vi "ex_GetPacketData.vi"(0 "file refs":T1={"file ref"=refnum, "file size (bytes:0)"=0, "read pointer (bytes:0)"=0, "chunk size (bytes:65000)"=65000}, 1 "channel info in":T3[](array[typedef]) {"Delta X" format="%.2p"; "X0" format="%<%X\n%x>T"; "Timestamp" format="%<%X\n%x>T"}, 2 "first call?":bool=TRUE, 5 "current chunk":string, 7 "delimiter":string="\t", 9 "file_params":T2={"include col headings?"=TRUE, "x_columns"=0, "col headings always?"=TRUE, "time preference"=0, "hide col headings"=FALSE} {"time preference" items=["Absolute", "Relative"]; "x_columns" items=["None", "One", "Multiple"]}, 11 "error in (no error)":errorcluster, 12 "Decimal Separator":string) -> (3 "channel info out":T3[](array[typedef]) {"Delta X" format="%.2p"; "X0" format="%<%X\n%x>T"; "Timestamp" format="%<%X\n%x>T"}, 4 "dup file refs":T1={"file ref"=refnum, "file size (bytes:0)"=0, "read pointer (bytes:0)"=0, "chunk size (bytes:65000)"=65000}, 6 "chunk out":string, 8 "data":dbl[][](array[numeric]) format="%.2f", 10 "end-of-file?":bool, 14 "comment":string, 15 "error out":errorcluster)   [LabVIEW 2020]
uses:
  <vilib>/express/express input/ExFileReadBlock.llb/ex_ReadFileParams.ctl
  <vilib>/express/express shared/ExFile.llb/ex_AllChanInfo.ctl
  <vilib>/express/express shared/ExFile.llb/ex_FileReference.ctl
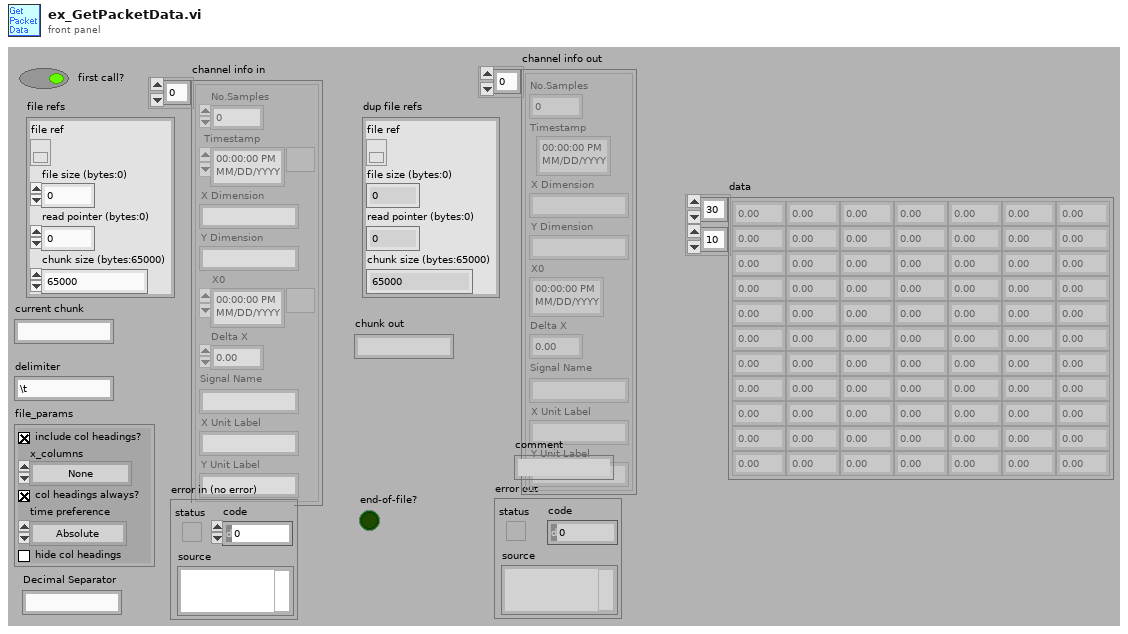
[diagram p1: front panel]
types:
  T1 = typedef "ex_FileReference.ctl" = cluster{"file ref":refnum<file>, "file size (bytes:0)":i32, "read pointer (bytes:0)":i32, "chunk size (bytes:65000)":i32}
  T2 = typedef "ex_ReadFileParams.ctl" = cluster{"include col headings?":bool, "x_columns":u16, "col headings always?":bool, "time preference":u16, "hide col headings":bool}
  T3 = typedef "ex_AllChanInfo.ctl" = cluster{"No.Samples":i32, "Timestamp":timestamp, "X Dimension":string, "Y Dimension":string, "X0":timestamp, "Delta X":dbl, "Signal Name":string, "X Unit Label":string, "Y Unit Label":string}
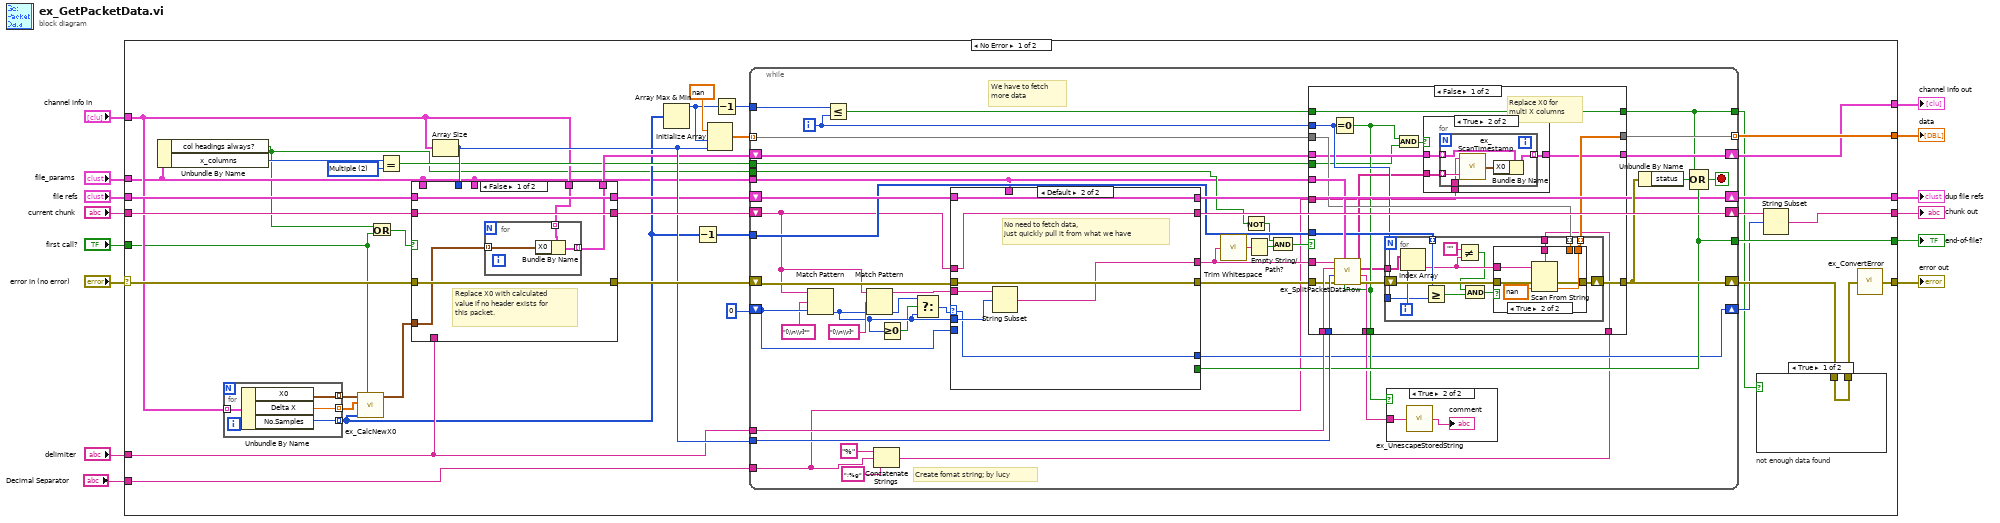
[diagram p0: block diagram]
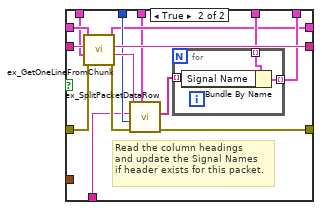
[diagram p2: hidden frame]
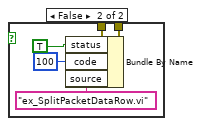
[diagram p3: hidden frame]
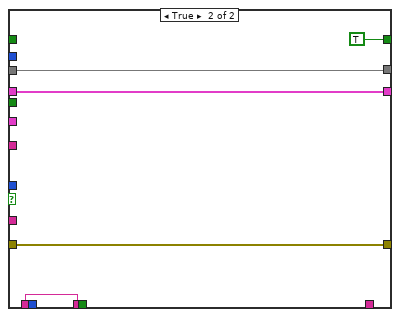
[diagram p6: hidden frame]
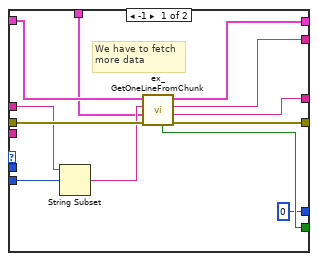
[diagram p7: hidden frame]
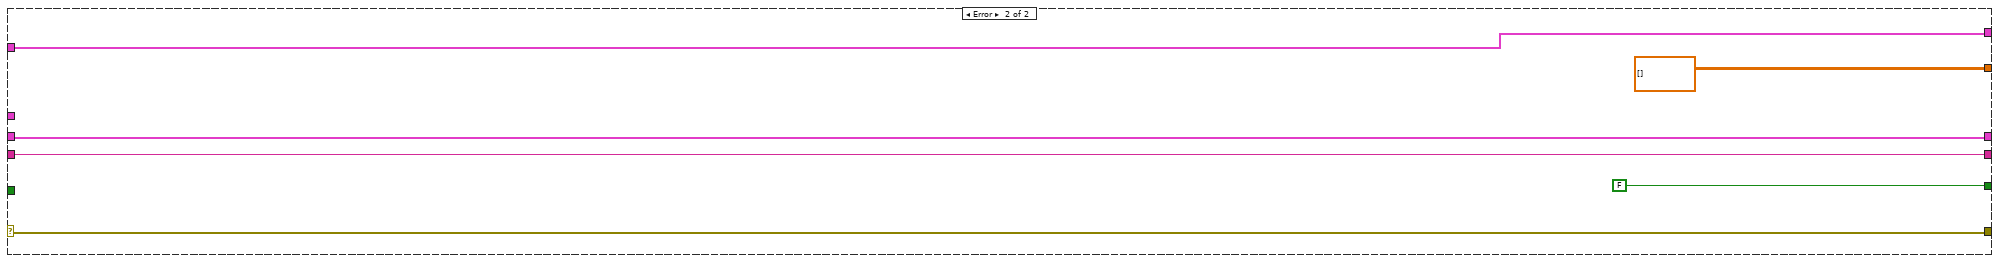
[diagram p9: hidden frame]
diagram:
  n1 = case shown="No Error" "error in (no error)" {
    selector: "error in (no error)" -> [w44 w219]
    tunnel: "current chunk" -> [w45 w220]
    tunnel: [w24 w220] -> w12
    tunnel: [w46 w219] -> w11
    tunnel: [w48 dbl[][] []] -> w10
    tunnel: [w47 FALSE] -> w9
    tunnel: "channel info in" -> [w29 w216]
    tunnel: [w33 w216] -> w7
    tunnel: "file refs" -> [w35 w215]
    tunnel: [w37 w215] -> w5
    tunnel: "delimiter" -> [w36 _]
    tunnel: "file_params" -> [w21 _]
    tunnel: "first call?" -> [w19 _]
    tunnel: "Decimal Separator" -> [w17 _]
    frame No Error {
      w32 = u16 2 items=["None", "One", "Multiple"] ("x_columns")
      n2 = Unbundle By Name(w21) -> ("col headings always?"=w20:bool, "x_columns"=w30:u16)
      n3 = for {
        tunnel: w29 -> [w57] mode=indexing
        tunnel: [w56] -> w16 mode=indexing
        tunnel: [w55] -> w23 mode=indexing
        tunnel: [w54] -> w15 mode=indexing
        n4 = Unbundle By Name(w57) -> ("X0"=w54:timestamp, "Delta X"=w56:dbl, "No.Samples"=w55:i32)
      }
      n5 = call <vilib>:"ex_CalcNewX0.vi"("reset"=w19, "samples"=w23, "Delta X"=w16, "Initial X0"=w15) -> ("X0"=w28:timestamp[])  [unwired: 7 out]
      n6 = Or(x=w20, y=w19) -> (x .or. y?=w18:bool)
      n7 = Equal?(x=w30, y=w32) -> (x = y?=w31:bool)
      n8 = Array Size(array=w29) -> (size(s)=w41:i32)
      n9 = case shown="False" w18 {
        tunnel: w45 -> [w62 w81]
        tunnel: w44 -> [w61 w80]
        tunnel: w35 -> [w63 w79]
        tunnel: [w62 w78] -> w43
        tunnel: [w61 w75] -> w42
        tunnel: [w59 w74] -> w34
        tunnel: w29 -> [w60 w72]
        tunnel: w41 -> [_ w71]
        tunnel: [w63 w70] -> w38
        tunnel: w36 -> [_ w69]
        tunnel: w21 -> [_ w68]
        tunnel: w28 -> [w58 _]
        tunnel: w21 -> [_ w67]
        frame False {
          # "Replace X0 with calculated \nvalue if no header exists for \nthis packet."
          n10 = for {
            tunnel: w60 -> [w66] mode=indexing
            tunnel: [w65] -> w59 mode=indexing
            tunnel: w58 -> [w64] mode=indexing
            n11 = Bundle By Name(cluster=w66, "X0"=w64) -> (w65:T3)
          }
        }
        frame True {
          # "Read the column headings \nand update the Signal Names \nif header exists for this packet."
          n12 = call <vilib>:"ex_GetOneLineFromChunk.vi"("error in (no error)"=w80, "file_params"=w67, "current chunk"=w81, "file refs in"=w79) -> ("error out"=w76:errorcluster, "line"=w77:string, "chunk out"=w78:string, "dup file refs"=w70:T1)  [unwired: 4 out]
          n13 = call <vilib>:"ex_SplitPacketDataRow.vi"("file_params"=w68, "error in (no error)"=w76, "nChannels"=w71, "delimiter"=w69, "row"=w77) -> ("error out"=w75:errorcluster, "y strings"=w73:string[])  [unwired: 1 in, 4 out]
          n14 = for {
            tunnel: w72 -> [w84] mode=indexing
            tunnel: [w83] -> w74 mode=indexing
            tunnel: w73 -> [w82] mode=indexing
            n15 = Bundle By Name(cluster=w84, "Signal Name"=w82) -> (w83:T3)
          }
        }
      }
      n16 = Array Max & Min(array=w23) -> (max value=w51:i32)  [unwired: 3 out]
      n17 = Decrement(x=w23) -> (x-1=w49:i32[])
      n18 = Initialize Array(nan ("element"), w51, w41) -> (w50:dbl[][])
      n19 = Decrement(x=w51) -> (x-1=w53:i32)
      n20 = while {
        shift-right: [w132] -> w26
        shift-left: w43 -> [w106]
        tunnel: w53 -> [w134]
        tunnel: w50 -> [w122] mode=indexing
        shift-right: [w129] -> w39
        shift-left: w42 -> [w133]
        tunnel: w49 -> [w123]
        tunnel: [w121] -> w48 mode=indexing
        tunnel: [w126] -> w47
        tunnel: w21 -> [w95]
        tunnel: w36 -> [w131]
        tunnel: w41 -> [w130]
        tunnel: [w97] -> w22
        shift-right: [w124] -> w37
        shift-left: w38 -> [w125]
        shift-right: [w118] -> w33
        shift-left: w34 -> [w119]
        tunnel: w31 -> [w101]
        shift-right: [w115] -> w25
        shift-left: 0 -> [w113]
        tunnel: w20 -> [w99]
        tunnel: w17 -> [w91]
        i -> [w120]
        stop <- w127 stop-if-true
        # "Create fomat string; by lucy"
        # "We have to fetch\nmore data"
        n21 = Match Pattern(string=w106, regular expression="[\\n\\r]*", offset (0)=w113) -> (offset past match=w109:i32)  [unwired: 3 out]
        n22 = Less Or Equal?(x=w134, y=w120) -> (x <= y?=w98:bool)
        n23 = Match Pattern(string=w106, regular expression="[\\n\\r]", offset (0)=w109) -> (before substring=w114:string, offset past match=w110:i32)  [unwired: 2 out]
        n24 = Concatenate Strings("%" ("string"), w91, ";%g" ("string")) -> (w92:string)
        n25 = Greater Or Equal To 0?(x=w109) -> (x >= 0?=w108:bool)
        n26 = Select(t=w110, s=w108, f=w109) -> (s? t:f=w105:i32)
        n27 = case shown="Default" w105 {
          selector: w105 -> [_ w206]
          tunnel: w133 -> [w205 w211]
          tunnel: w106 -> [w197 w210]
          tunnel: [w204 w211] -> w107
          tunnel: [w203 w207] -> w103
          tunnel: [w202 w210] -> w132
          tunnel: [w201 _] -> w126
          tunnel: w125 -> [w200 w212]
          tunnel: [w199 w212] -> w124
          tunnel: [0 ("offset past match") w206] -> w115
          tunnel: w113 -> [w195 _]
          tunnel: w114 -> [_ w209]
          tunnel: w109 -> [_ w208]
          tunnel: w95 -> [w194 _]
          frame -1 {
            # "We have to fetch\nmore data"
            n28 = String Subset(string=w197, offset (0)=w195) -> (substring=w196:string)  [unwired: 1 out]
            n29 = call <vilib>:"ex_GetOneLineFromChunk.vi"("error in (no error)"=w205, "file_params"=w194, "current chunk"=w196, "file refs in"=w200) -> ("error out"=w204:errorcluster, "line"=w203:string, "chunk out"=w202:string, "dup file refs"=w199:T1, "end-of-file?"=w201:bool)  [unwired: 3 out]
          }
          frame Default {
            # "No need to fetch data,\njust quickly pull it from what we have"
            n30 = String Subset(string=w209, offset (0)=w208) -> (substring=w207:string)  [unwired: 1 out]
          }
        }
        n31 = call <vilib>:"Trim Whitespace.vi"("string"=w103) -> ("trimmed string"=w104:string)  [unwired: 1 in]
        n32 = Not(x=w99) -> (.not. x?=w100:bool)
        n33 = Empty String/Path?(string/path=w104) -> (empty?=w102:bool)
        n34 = And(x=w100, y=w102) -> (x .and. y?=w96:bool)
        n35 = case shown="False" w96 {
          tunnel: w95 -> [w156 _]
          tunnel: w131 -> [w155 w193]
          tunnel: w130 -> [w154 _]
          tunnel: [w152 w192] -> w129
          tunnel: w123 -> [w151 _]
          tunnel: w122 -> [w150 w191]
          tunnel: [w149 w191] -> w121
          tunnel: w120 -> [w148 _]
          tunnel: w119 -> [w146 w190]
          tunnel: [w145 w190] -> w118
          tunnel: [w143 w193] -> w117
          tunnel: [w142 _] -> w116
          tunnel: w107 -> [w140 w192]
          tunnel: w103 -> [w139 _]
          tunnel: w101 -> [w138 _]
          tunnel: w98 -> [w137 _]
          tunnel: [w137 TRUE] -> w97
          tunnel: w92 -> [w136 _]
          tunnel: w91 -> [w135 _]
          frame False {
            # "Replace X0 for\nmulti X columns"
            n36 = Equal To 0?(x=w148) -> (x = 0?=w142:bool)
            n37 = call <vilib>:"ex_SplitPacketDataRow.vi"("get additional item"=w142, "file_params"=w156, "error in (no error)"=w140, "nChannels"=w154, "delimiter"=w155, "row"=w139) -> ("error out"=w153:errorcluster, "additional item"=w143:string, "y strings"=w141:string[], "x strings"=w144:string[])  [unwired: 2 out]
            n38 = for {
              shift-right: [w180] -> w152
              shift-left: w153 -> [w176]
              tunnel: w136 -> [w179]
              tunnel: w150 -> [w178] mode=indexing
              tunnel: w151 -> [w174] mode=indexing
              tunnel: [w177] -> w149 mode=indexing
              tunnel: w141 -> [w175]
              tunnel: w148 -> [w172]
              i -> [w173]
              n39 = Index Array(array=w175, index=w173) -> (element=w171:string)
              n40 = Greater Or Equal?(x=w174, y=w172) -> (x >= y?=w169:bool)
              n41 = Not Equal?(x="", y=w171) -> (x != y?=w167:bool)
              n42 = And(x=w167, y=w169) -> (x .and. y?=w168:bool)
              n43 = case shown="True" w168 {
                tunnel: w176 -> [w181 w188]
                tunnel: w179 -> [_ w187]
                tunnel: w171 -> [_ w186]
                tunnel: w178 -> [w182 _]
                tunnel: [w182 w184] -> w177
                tunnel: [w181 w183] -> w180
                frame False {
                }
                frame True {
                  n44 = Scan From String(format string=w187, input string=w186, error in=w188, default 1=nan ("default value 1")) -> (error out=w183:errorcluster, output 1=w184:dbl)  [unwired: 1 in, 2 out]
                }
              }
            }
            n45 = And(x=w142, y=w138) -> (x .and. y?=w147:bool)
            n46 = case shown="True" w147 {
              tunnel: w146 -> [w157 w161]
              tunnel: [w157 w159] -> w145
              tunnel: w144 -> [_ w160]
              tunnel: w135 -> [_ w158]
              frame False {
              }
              frame True {
                n47 = for {
                  tunnel: w161 -> [w166] mode=indexing
                  tunnel: w160 -> [w164] mode=indexing
                  tunnel: [w165] -> w159 mode=indexing
                  tunnel: w158 -> [w162]
                  n48 = call <vilib>:"ex_ScanTimestamp.vi"("High-Precision Numeric String"=w164, "Decimal point"=w162) -> ("High-Precision Numeric"=w163:timestamp)  [unwired: 1 in, 2 out]
                  n49 = Bundle By Name(cluster=w166, "X0"=w163) -> (w165:T3)
                }
              }
            }
          }
          frame True {
          }
        }
        n50 = case shown="True" w116 {
          tunnel: w117 -> [_ w214]
          frame False {
          }
          frame True {
            n51 = call <vilib>:"ex_UnescapeStoredString.vi"("stored string"=w214) -> ("parsed string"=→"comment":string)
          }
        }
        n52 = Unbundle By Name(w129) -> ("status"=w128:bool)
        n53 = Compound Arithmetic op=OR(w97, w128, w126) -> (w127:bool)
      }
      n54 = case "not enough data found" shown="True" w22 {
        tunnel: w39 -> [w85 w90]
        tunnel: [w85 w87] -> w40
        frame True {
        }
        frame False {
          n55 = Bundle By Name(cluster=w90, "status"=TRUE, "code"=100, "source"="ex_SplitPacketDataRow.vi") -> (w87:errorcluster)
        }
      }
      n56 = String Subset(string=w26, offset (0)=w25) -> (substring=w24:string)  [unwired: 1 out]
      n57 = call <vilib>:"ex_ConvertError.vi"("error in (no error)"=w40) -> ("error out"=w46:errorcluster)  [unwired: 4 out]
    }
    frame Error {
    }
  }
  "end-of-file?" <- w9
  "error out" <- w11
  "data" <- w10
  "chunk out" <- w12
  "channel info out" <- w7
  "dup file refs" <- w5
